vi "test_Format Debug String_All inputs have unusual chars.vi"(8 "error in (no error)":errorcluster, 11 "TestCase in":refnum<class "Instrument Addon Unit Tests.lvclass">) -> (0 "error out":errorcluster, 3 "TestCase out":refnum<class "Instrument Addon Unit Tests.lvclass">)   [LabVIEW 2018, in "Instrument Addon Unit Tests.lvclass"]
uses:
  Instrument Addon Unit Tests.lvclass
  <vilib>/addons/_JKI Toolkits/VI Tester/TestCase.llb/TestCase.lvclass
  Addon/Addon Engine/Instrument Addon Engine.lvlib
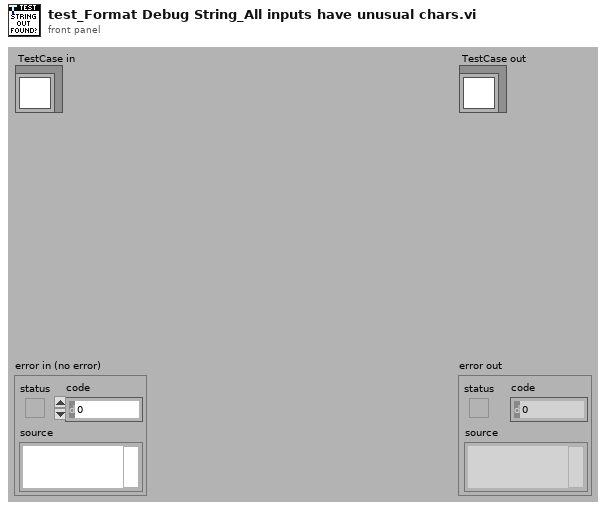
[diagram p1: front panel]
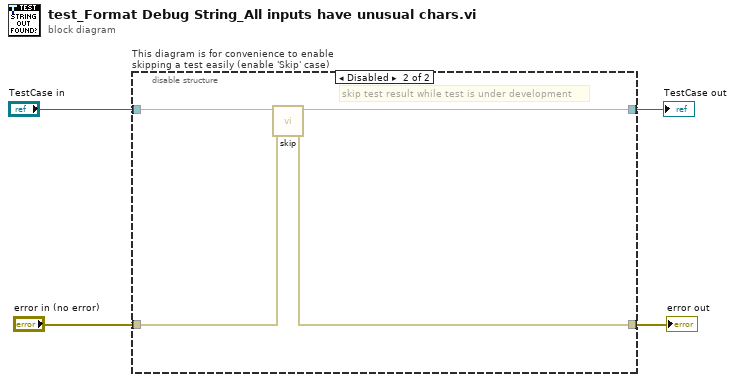
[diagram p0: block diagram]
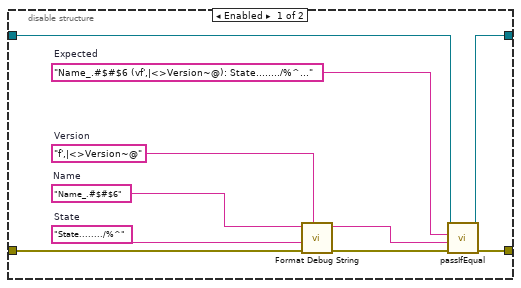
[diagram p2: hidden frame]
diagram:
  n1 = disable-structure "This diagram is for convenience to enable skipping a test easily (enable 'Skip' case)" shown="Disabled" {
    disable-tunnel: "TestCase in" -> [w12 w18]
    disable-tunnel: [w13 w16] -> w1
    disable-tunnel: [w14 w17] -> w3
    disable-tunnel: "error in (no error)" -> [w11 w15]
    frame Enabled {
      w6 = "State......../%^"  # State
      w7 = "Name_.#$#$6"  # Name
      w8 = "f',|<>Version~@"  # Version
      w9 = "Name_.#$#$6 (vf',|<>Version~@): State......../%^..."  # Expected
      n2 = call "Format Debug String.vi"("Version"=w8, "error in (no error)"=w11, "State"=w6, "Name"=w7) -> ("error out"=w10:errorcluster, "Debug String"=w5:string)  [unwired: 6 in]
      n3 = call-dynamic "passIfEqual.vi"("error in (no error)"=w10, "y"=w5, "x"=w9, "TestCase in"=w12) -> ("error out"=w14:errorcluster, "TestCase out"=w13:refnum<class "Instrument Addon Unit Tests.lvclass">)  [unwired: 6 in]
    }
    frame Disabled {
      # "skip test result while test is under development"
      n4 = call <vilib>:"skip.vi"("error in (no error)"=w15, "TestCase in"=w18) -> ("error out"=w17:errorcluster, "TestCase out"=w16:refnum<class "Instrument Addon Unit Tests.lvclass">)  [unwired: 8 in]
    }
  }
  "error out" <- w3
  "TestCase out" <- w1
